vi "题目3测量温度子VI.vi"(0 "停止":bool, 2 "温度单位":bool) -> (1 "温度计":dbl(slide) scale=0.0..100.0, 3 "温度":string)   [LabVIEW 2017]
panel:
  # "℉"
  # "℃"
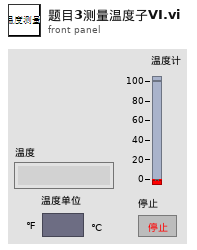
[diagram p1: front panel]
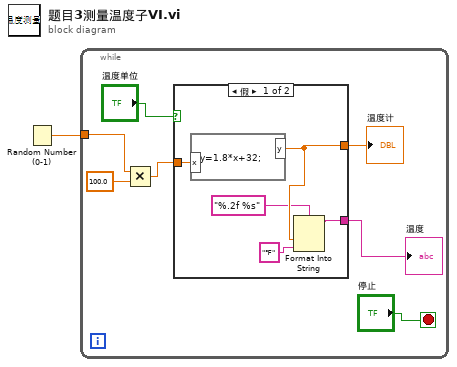
[diagram p0: block diagram]
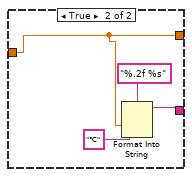
[diagram p2: hidden frame]
diagram:
  n1 = Random Number (0-1)() -> (number: 0 to 1=w1:dbl)
  n2 = while {
    tunnel: w1 -> [w5]
    stop <- "停止" stop-if-true
    n3 = Multiply(x=w5, y=100.0) -> (x*y=w6:dbl)
    n4 = case shown="假" "温度单位" {
      tunnel: [w10 w16] -> w7
      tunnel: w6 -> [w13 w16]
      tunnel: [w12 w15] -> w2
      frame False {
        n5 = formula code="y=1.8*x+32;"("x"=w13) -> ("y"=w10:dbl)
        n6 = Format Into String(format string="%.2f %s" ("格式字符串"), w10, "℉") -> (resulting string=w12:string)  [unwired: 2 in, 1 out]
      }
      frame True {
        n7 = Format Into String(format string="%.2f %s" ("格式字符串"), w16, "℃") -> (resulting string=w15:string)  [unwired: 2 in, 1 out]
      }
    }
    "温度计" <- w7
    "温度" <- w2
  }
